vi "HFRR ADV v026 new software.vi"() -> ()   [LabVIEW 2025] (continued)
        n321 = Equal?(x=w400, y="Service@123") -> (x = y?=w401:bool)
        n322 = case shown="False" w401 {
          selector: w401 -> [w405 w407]
          frame False {
            n323 = local write "Service Password enable"(w405) -> ()
            n324 = property on="Service Password Log" class="Str"("Visible"=TRUE) -> ()  [unwired: 2 in, 2 out]
          }
          frame True {
            n325 = property on="Service Password Log" class="Str"("Visible"=FALSE) -> ()  [unwired: 2 in, 2 out]
            "Service Password enable" <- w407
          }
        }
      }
      event "Sign In": Value Change {
        w409 = FALSE ("Visible")
        n326 = event-data() -> ()  [unwired: 1 in, 6 out]
        n327 = property on="About" class="Clust (strict)"("Visible"=w409) -> ()  [unwired: 2 in, 2 out]
        n328 = property on="Password 3" class="Clust (strict)"("Visible"=w409) -> ()  [unwired: 2 in, 2 out]
        n329 = property on="Service Password Log" class="Str"("Visible"=FALSE) -> ()  [unwired: 2 in, 2 out]
      }
      event "Info": Value Change {
        n330 = event-data() -> ()  [unwired: 1 in, 6 out]
        n331 = local read "Info"() -> (w411:bool)
        n332 = case shown="False" w411 {
          frame False {
            n333 = property on="About" class="Clust (strict)"("Visible"=FALSE) -> ()  [unwired: 2 in, 2 out]
          }
          frame True {
            n334 = property on="About" class="Clust (strict)"("Visible"=TRUE) -> ()  [unwired: 2 in, 2 out]
          }
        }
      }
      event "Calibration": Value Change {
        n335 = event-data() -> ()  [unwired: 1 in, 6 out]
        n336 = local read "Calibration"() -> (w415:bool)
        n337 = case shown="False" w415 {
          frame False {
            n338 = property on="Calibration 2" class="TabCtl (strict)"("Visible"=FALSE) -> ()  [unwired: 2 in, 2 out]
            n339 = local write "Cal Password"("" ("Cal Password")) -> ()
          }
          frame True {
            n340 = property on="Calibration 2" class="TabCtl (strict)"("Visible"=TRUE) -> ()  [unwired: 2 in, 2 out]
            n341 = local write "Cal Password"("" ("Cal Password")) -> ()
          }
        }
        n342 = property on="Wrong Password" class="Str"("Visible"=FALSE) -> ()  [unwired: 2 in, 2 out]
      }
      event "Cal Password": Value Change {
        n343 = event-data() -> ()  [unwired: 1 in, 6 out]
        n344 = local read "Cal Password"() -> (w423:string)
        n345 = call <vilib>:"Trim Whitespace.vi"("string"=w423) -> ("trimmed string"=w422:string)  [unwired: 1 in]
        n346 = Equal?(x=w422, y="Cal@321") -> (x = y?=w420:bool)
        n347 = case shown="True" w420 {
          frame False {
            n348 = property on="Wrong Password" class="Str"("Visible"=TRUE) -> ()  [unwired: 2 in, 2 out]
          }
          frame True {
            n349 = property on="Wrong Password" class="Str"("Visible"=FALSE) -> ()  [unwired: 2 in, 2 out]
            n350 = local write "Main Tab"(T2."About" ("Main Tab")) -> ()
            n351 = local write "Cal Password"("" ("Cal Password")) -> ()
            n352 = local write "Main Dashboard Buttons"(T1."About" ("Main Dashboard Buttons")) -> ()
            n353 = property on="Calibration 2" class="TabCtl (strict)"("Visible"=FALSE) -> ()  [unwired: 2 in, 2 out]
            n354 = local write "Calibration"(FALSE ("Calibration")) -> ()
          }
        }
      }
      event "Calibration Selection": Value Change {
        n355 = event-data() -> ()  [unwired: 1 in, 6 out]
        n356 = local read "Calibration Selection"() -> (w432:T8)
        n357 = case shown="\"Stroke Calibration\"" w432 {
          tunnel: [T7."Stroke" ("Main Calibration Tab") T7."Friction" ("Main Calibration Tab") T7."Main" ("Main Calibration Tab") T7."Temperature" ("Main Calibration Tab")] -> w431
          frame "Stroke Calibration" {
          }
          frame "Friction Force Calibration" {
          }
          frame Default {
          }
          frame "Temperature Calibration" {
          }
        }
        n358 = local write "Main Calibration Tab"(w431) -> ()
      }
      event "Back Stroke": Value Change {
        n359 = event-data() -> ()  [unwired: 1 in, 6 out]
        n360 = local write "Main Stroke Tab"(T9."Step 1" ("Main Stroke Tab")) -> ()
        n361 = local write "Main Calibration Tab"(T7."Main" ("Main Calibration Tab")) -> ()
        n362 = local write "Back Stroke"(FALSE ("Back Stroke")) -> ()
      }
      event "Step 2 Back": Value Change {
        n363 = event-data() -> ()  [unwired: 1 in, 6 out]
        n364 = local write "Main Stroke Tab"(T9."Step 1" ("Main Stroke Tab")) -> ()
        n365 = local write "Step 2 Back"(FALSE ("Back Stroke")) -> ()
      }
      event "Step 3 Back": Value Change {
        n366 = event-data() -> ()  [unwired: 1 in, 6 out]
        n367 = local write "Main Stroke Tab"(T9."Step 2" ("Main Stroke Tab")) -> ()
        n368 = local write "Step 3 Back"(FALSE ("Back Stroke")) -> ()
      }
      event "Step 4 Back": Value Change {
        n369 = event-data() -> ()  [unwired: 1 in, 6 out]
        n370 = local write "Main Stroke Tab"(T9."Step 3" ("Main Stroke Tab")) -> ()
        n371 = local write "Step 4 Back"(FALSE ("Back Stroke")) -> ()
      }
      event "Step 5 Back": Value Change {
        n372 = event-data() -> ()  [unwired: 1 in, 6 out]
        n373 = local write "Main Stroke Tab"(T9."Step 4" ("Main Stroke Tab")) -> ()
        n374 = local write "Step 5 Back"(FALSE ("Back Stroke")) -> ()
      }
      event "Step 6 Back": Value Change {
        n375 = event-data() -> ()  [unwired: 1 in, 6 out]
        n376 = local write "Main Stroke Tab"(T9."Step 5" ("Main Stroke Tab")) -> ()
        n377 = local write "Step 6 Back"(FALSE ("Back Stroke")) -> ()
      }
      event "Back Stroke step 7": Value Change {
        n378 = event-data() -> ()  [unwired: 1 in, 6 out]
        n379 = local write "Main Stroke Tab"(T9."Step 6" ("Main Stroke Tab")) -> ()
        n380 = local write "Back Stroke step 7"(FALSE ("Back Stroke")) -> ()
      }
      event "Back Stroke step 8": Value Change {
        n381 = event-data() -> ()  [unwired: 1 in, 6 out]
        n382 = local write "Main Stroke Tab"(T9."Step 7" ("Main Stroke Tab")) -> ()
        n383 = local write "Back Stroke step 8"(FALSE ("Back Stroke")) -> ()
      }
      event "Back Stroke 8": Value Change {
        n384 = event-data() -> ()  [unwired: 1 in, 6 out]
        n385 = local write "MOVE CARRIAGE TO"(0.2 ("MOVE CARRIAGE TO")) -> ()
        n386 = local write "Main Stroke Tab"(T9."Step 1" ("Main Stroke Tab")) -> ()
        n387 = local write "Back Stroke 8"(FALSE ("Back Stroke 8")) -> ()
      }
      event "Continue Stroke": Value Change {
        n388 = event-data() -> ()  [unwired: 1 in, 6 out]
        n389 = local write "Main Stroke Tab"(T9."Step 2" ("Main Stroke Tab")) -> ()
        n390 = local write "Continue Stroke"(FALSE ("Continue Stroke")) -> ()
      }
      event "Continue Stroke step 2": Value Change {
        n391 = event-data() -> ()  [unwired: 1 in, 6 out]
        n392 = local write "Main Stroke Tab"(T9."Step 3" ("Main Stroke Tab")) -> ()
        n393 = local write "Continue Stroke step 2"(FALSE ("Continue Stroke")) -> ()
      }
      event "Continue Stroke step 3": Value Change {
        n394 = event-data() -> ()  [unwired: 1 in, 6 out]
        n395 = local write "Main Stroke Tab"(T9."Step 4" ("Main Stroke Tab")) -> ()
        n396 = local write "Continue Stroke step 3"(FALSE ("Continue Stroke")) -> ()
      }
      event "Continue Stroke step 4": Value Change {
        n397 = event-data() -> ()  [unwired: 1 in, 6 out]
        n398 = local write "Main Stroke Tab"(T9."Step 5" ("Main Stroke Tab")) -> ()
        n399 = local write "Continue Stroke step 4"(FALSE ("Continue Stroke")) -> ()
      }
      event "Continue Stroke step 5": Value Change {
        n400 = event-data() -> ()  [unwired: 1 in, 6 out]
        n401 = local write "Main Stroke Tab"(T9."Step 6" ("Main Stroke Tab")) -> ()
        n402 = local write "Continue Stroke step 5"(FALSE ("Continue Stroke")) -> ()
      }
      event "Continue Stroke step 6": Value Change {
        n403 = event-data() -> ()  [unwired: 1 in, 6 out]
        n404 = local write "Main Stroke Tab"(T9."Step 7" ("Main Stroke Tab")) -> ()
        n405 = local write "Continue Stroke step 6"(FALSE ("Continue Stroke")) -> ()
      }
      event "Continue Stroke step 7": Value Change {
        w471 = FALSE ("0.2mm")
        n406 = event-data() -> ()  [unwired: 1 in, 6 out]
        n407 = local write "0.4 mm"(w471) -> ()
        n408 = local write "0.6 mm"(w471) -> ()
        n409 = local write "1.0 mm"(w471) -> ()
        n410 = local write "1.2 mm"(w471) -> ()
        n411 = local write "0.2 2"(w471) -> ()
        n412 = local write "0.4 2"(w471) -> ()
        n413 = local write "0.6 2"(w471) -> ()
        n414 = local write "0.8 2"(w471) -> ()
        n415 = local write "1.0 2"(w471) -> ()
        n416 = local write "1.2"(w471) -> ()
        n417 = local write "0.2mm"(w471) -> ()
        n418 = local write "0.8mm"(w471) -> ()
        n419 = local write "Main Stroke Tab"(T9."Step 8" ("Main Stroke Tab")) -> ()
        n420 = local write "Continue Stroke step 7"(FALSE ("Continue Stroke")) -> ()
        n421 = local write "Stroke Test Complete"(T10."Test Progress" ("Stroke Test Complete")) -> ()
        "Position Measurment Temp" <- 0.0 ("Position Measurment Temp")
        "Calibration Tare" <- TRUE ("Calibration Tare")
        "MOVE CARRIAGE TO" <- 0.2 ("MOVE CARRIAGE TO")
      }
      event "Continue Stroke step 8": Value Change {
        n422 = event-data() -> ()  [unwired: 1 in, 6 out]
        n423 = local read "LVDT STROKE  Calibration"() -> (w476:dbl)
        n424 = local read "Position Measurment Temp"() -> (w477:dbl)
        n425 = case shown="7" w477 {
          selector: w477 -> [w482 w487 w492 w497 w502 w506 w509 w510]
          tunnel: w476 -> [w478 w483 w488 w493 w498 w503 _ _]
          frame 0, Default {
            w480 = TRUE ("0.2mm")
            n426 = Increment(x=w482) -> (x+1=w481:i32)
            n427 = local write "Position Measurment Temp"(w481) -> ()
            n428 = local write "0.2mm"(w480) -> ()
            n429 = local write "0.2 2"(w480) -> ()
            n430 = local write "MOVE CARRIAGE TO"(0.4 ("MOVE CARRIAGE TO")) -> ()
            "Calibration 0.2" <- w478
          }
          frame 1 {
            w485 = TRUE ("0.4 mm")
            n431 = Increment(x=w487) -> (x+1=w486:i32)
            n432 = local write "Calibration 0.4"(w483) -> ()
            n433 = local write "Position Measurment Temp"(w486) -> ()
            n434 = local write "0.4 mm"(w485) -> ()
            n435 = local write "MOVE CARRIAGE TO"(0.6 ("MOVE CARRIAGE TO")) -> ()
            n436 = local write "0.4 2"(w485) -> ()
          }
          frame 2 {
            w490 = TRUE ("0.6 mm")
            n437 = Increment(x=w492) -> (x+1=w491:i32)
            n438 = local write "Calibration 0.6"(w488) -> ()
            n439 = local write "Position Measurment Temp"(w491) -> ()
            n440 = local write "0.6 2"(w490) -> ()
            n441 = local write "0.6 mm"(w490) -> ()
            n442 = local write "MOVE CARRIAGE TO"(0.8 ("MOVE CARRIAGE TO")) -> ()
          }
          frame 3 {
            w494 = TRUE ("0.6 mm")
            n443 = Increment(x=w497) -> (x+1=w496:i32)
            n444 = local write "Position Measurment Temp"(w496) -> ()
            n445 = local write "MOVE CARRIAGE TO"(1.0 ("MOVE CARRIAGE TO")) -> ()
            n446 = local write "0.8mm"(w494) -> ()
            n447 = local write "0.8 2"(w494) -> ()
            "Calibration 0.8" <- w493
          }
          frame 4 {
            w499 = TRUE ("0.6 mm")
            n448 = Increment(x=w502) -> (x+1=w501:i32)
            n449 = local write "Position Measurment Temp"(w501) -> ()
            n450 = local write "MOVE CARRIAGE TO"(1.2 ("MOVE CARRIAGE TO")) -> ()
            n451 = local write "1.0 mm"(w499) -> ()
            n452 = local write "1.0 2"(w499) -> ()
            "Calibration 1.0" <- w498
          }
          frame 5 {
            w504 = TRUE ("0.6 mm")
            n453 = Increment(x=w506) -> (x+1=w505:i32)
            n454 = local write "Position Measurment Temp"(w505) -> ()
            n455 = local write "1.2 mm"(w504) -> ()
            n456 = local write "1.2"(w504) -> ()
            "Calibration 1.2" <- w503
          }
          frame 6 {
            n457 = Increment(x=w509) -> (x+1=w508:i32)
            n458 = local write "Position Measurment Temp"(w508) -> ()
            n459 = local write "Stroke Test Complete"(T10."Stroke Points Completed" ("Stroke Test Complete")) -> ()
          }
          frame 7 {
            n460 = stacked-sequence {
              tunnel: w510 -> [w511 _ _]
              frame #0 {
                n461 = Increment(x=w511) -> (x+1=w512:i32)
                n462 = local write "Main Stroke Tab"(T9."Step 9" ("Main Stroke Tab")) -> ()
                n463 = local write "Position Measurment Temp"(w512) -> ()
                n464 = Insert Into Array(array=dbl[] [], new element #1=0.2 ("new element/subarray"), new element #2=0.4 ("new element/subarray"), new element #3=0.6 ("new element/subarray"), new element #4=0.8 ("new element/subarray"), new element #5=1.0 ("new element/subarray"), new element #6=1.2 ("new element/subarray")) -> (→"1D stroke":dbl[])  [unwired: 1 in]
                n465 = local read "Calibration 0.2"() -> (w519:dbl)
                n466 = local read "Calibration 0.4"() -> (w518:dbl)
                n467 = local read "Calibration 0.6"() -> (w517:dbl)
                n468 = local read "Calibration 0.8"() -> (w516:dbl)
                n469 = local read "Calibration 1.0"() -> (w515:dbl)
                n470 = local read "Calibration 1.2"() -> (w514:dbl)
                n471 = Insert Into Array(array=dbl[] [], new element #1=w519, new element #2=w518, new element #3=w517, new element #4=w516, new element #5=w515, new element #6=w514) -> (→"Calibrated Voltage Value":dbl[])  [unwired: 1 in]
              }
              frame #1 {
                n472 = local read "calibration values"() -> (w542:dbl[])
                n473 = local read "Calibrated Voltage Value"() -> (w544:dbl[])
                n474 = Index Array(array=w542, index #1=1 ("index"), index #2=3 ("index"), index #3=5 ("index"), index #4=7 ("index"), index #5=9 ("index"), index #6=11 ("index")) -> (element #1=w535:dbl, element #2=w534:dbl, element #3=w533:dbl, element #4=w532:dbl, element #5=w531:dbl, element #6=w530:dbl)
                n475 = local read "1D stroke"() -> (w545:dbl[])
                n476 = for {
                  tunnel: [w554] -> w543 mode=indexing
                  tunnel: w545 -> [w553] mode=indexing
                  tunnel: w544 -> [w552] mode=indexing
                  tunnel: w535 -> [w551]
                  tunnel: w534 -> [w550]
                  tunnel: w533 -> [w549]
                  tunnel: w532 -> [w548]
                  tunnel: w531 -> [w547]
                  tunnel: w530 -> [w546]
                  n477 = formula code="if (stroke == 0.2)\n{\n    if ((voltage >= REF_02 - 0.2) && (voltage <= REF_02 + 0.2))\n        status = 1;\n    else\n        status = 0;\n}\nelse if (stroke == 0.4)\n{\n    if ((voltage >= REF_04 - 0.2) && (voltage <= REF_04 + 0.2))\n        status = 1;\n    else\n        status = 0;\n}\nelse if (stroke == 0.6)\n{\n    if ((voltage >= REF_06 - 0.2) && (voltage <= REF_06 + 0.2))\n        status = 1;\n    else\n        status = 0;\n}\nelse if (stroke == 0.8)\n{\n    if ((voltage >= REF_08 - 0.2) && (voltage <= REF_08 + 0.2))\n        status = 1;\n    else\n        status = 0;\n}\nelse if (stroke == 1.0)\n{\n    if ((voltage >= REF_10 - 0.2) && (voltage <= REF_10 + 0.2))\n        status = 1;\n    else\n        status = 0;\n}\nelse if (stroke == 1.2)\n{\n    if ((voltage >= REF_12 - 0.2) && (voltage <= REF_12 + 0.2))\n        status = 1;\n    else\n        status = 0;\n}\nelse\n{\n    status = 0;\n}"("stroke"=w553, "voltage"=w552, "REF_02"=w551, "REF_04"=w550, "REF_06"=w549, "REF_08"=w548, "REF_10"=w547, "REF_12"=w546) -> ("status"=w554:dbl)
                }
                "Status" <- w543
              }
              frame #2 {
                w561 = 1.0
                n478 = local read "Status"() -> (w568:dbl[])
                n479 = Index Array(array=w568) -> (element #1=w567:dbl, element #2=w566:dbl, element #3=w565:dbl, element #4=w564:dbl, element #5=w563:dbl, element #6=w562:dbl)  [unwired: 6 in]
                n480 = Equal?(x=w566, y=w561) -> (x = y?=w559:bool)
                n481 = Equal?(x=w565, y=w561) -> (x = y?=w558:bool)
                n482 = Equal?(x=w564, y=w561) -> (x = y?=w557:bool)
                n483 = Equal?(x=w563, y=w561) -> (x = y?=w556:bool)
                n484 = Equal?(x=w562, y=w561) -> (x = y?=w555:bool)
                n485 = Equal?(x=w567, y=w561) -> (x = y?=w560:bool)
                n486 = case shown="True" w560 {
                  selector: w560 -> [w579 w580]
                  frame True {
                    n487 = local write "Point 1 - 0.2 mm"(w579) -> ()
                    n488 = property on="Point 1 - 0.2 mm" class="Bool"("Caption.Visible"=w579) -> ()  [unwired: 2 in, 2 out]
                  }
                  frame False {
                    n489 = local write "Point 1 - 0.2 mm"(w580) -> ()
                    n490 = property on="Point 1 - 0.2 mm" class="Bool"("Caption.Visible"=w580) -> ()  [unwired: 2 in, 2 out]
                  }
                }
                n491 = case shown="True" w559 {
                  selector: w559 -> [w577 w578]
                  frame True {
                    n492 = local write "Point 2 - 0.4 mm"(w577) -> ()
                    n493 = property on="Point 2 - 0.4 mm" class="Bool"("Caption.Visible"=w577) -> ()  [unwired: 2 in, 2 out]
                  }
                  frame False {
                    n494 = local write "Point 2 - 0.4 mm"(w578) -> ()
                    n495 = property on="Point 2 - 0.4 mm" class="Bool"("Caption.Visible"=w578) -> ()  [unwired: 2 in, 2 out]
                  }
                }
                n496 = case shown="True" w556 {
                  selector: w556 -> [w571 w572]
                  frame True {
                    n497 = local write "Point 5 - 1.0 mm"(w571) -> ()
                    n498 = property on="Point 5 - 1.0 mm" class="Bool"("Caption.Visible"=w571) -> ()  [unwired: 2 in, 2 out]
                  }
                  frame False {
                    n499 = local write "Point 5 - 1.0 mm"(w572) -> ()
                    n500 = property on="Point 5 - 1.0 mm" class="Bool"("Caption.Visible"=w572) -> ()  [unwired: 2 in, 2 out]
                  }
                }
                n501 = case shown="True" w558 {
                  selector: w558 -> [w575 w576]
                  frame True {
                    n502 = local write "Point 3 - 0.6 mm"(w575) -> ()
                    n503 = property on="Point 3 - 0.6 mm" class="Bool"("Caption.Visible"=w575) -> ()  [unwired: 2 in, 2 out]
                  }
                  frame False {
                    n504 = local write "Point 3 - 0.6 mm"(w576) -> ()
                    n505 = property on="Point 3 - 0.6 mm" class="Bool"("Caption.Visible"=w576) -> ()  [unwired: 2 in, 2 out]
                  }
                }
                n506 = case shown="True" w557 {
                  selector: w557 -> [w573 w574]
                  frame True {
                    n507 = local write "Point 4 - 0.8 mm"(w573) -> ()
                    n508 = property on="Point 4 - 0.8 mm" class="Bool"("Caption.Visible"=w573) -> ()  [unwired: 2 in, 2 out]
                  }
                  frame False {
                    n509 = local write "Point 4 - 0.8 mm"(w574) -> ()
                    n510 = property on="Point 4 - 0.8 mm" class="Bool"("Caption.Visible"=w574) -> ()  [unwired: 2 in, 2 out]
                  }
                }
                n511 = case shown="True" w555 {
                  selector: w555 -> [w569 w570]
                  frame True {
                    n512 = local write "Point 6 - 1.2 mm"(w569) -> ()
                    n513 = property on="Point 6 - 1.2 mm" class="Bool"("Caption.Visible"=w569) -> ()  [unwired: 2 in, 2 out]
                  }
                  frame False {
                    n514 = local write "Point 6 - 1.2 mm"(w570) -> ()
                    n515 = property on="Point 6 - 1.2 mm" class="Bool"("Caption.Visible"=w570) -> ()  [unwired: 2 in, 2 out]
                  }
                }
              }
            }
          }
        }
      }
      event "TEMPERATURE STEP Back 1", "TEMPERATURE STEP Back air Temp": Value Change {
        n516 = event-data() -> ()  [unwired: 1 in, 6 out]
        n517 = stacked-sequence {
          frame #0 {
            n518 = local write "Main Calibration Tab"(T7."Main" ("Main Calibration Tab")) -> ()
          }
          frame #1 {
            n519 = Wait (ms)(milliseconds to wait=u32 1000) -> ()  [unwired: 1 out]
          }
          frame #2 {
            n520 = local write "Due Write"("CAL;END" ("Command")) -> ()
          }
          frame #3 {
            n521 = Wait (ms)(milliseconds to wait=u32 2000) -> ()  [unwired: 1 out]
          }
          frame #4 {
            n522 = local write "Due Write"("CAL;END" ("Command")) -> ()
          }
        }
      }
      event "Temperature Continue Step 1": Value Change {
        n523 = event-data() -> ()  [unwired: 1 in, 6 out]
        n524 = stacked-sequence {
          frame #0 {
            n525 = Wait (ms)(milliseconds to wait=u32 1500) -> ()  [unwired: 1 out]
          }
          frame #1 {
            n526 = local write "Due Write"("CAL;START" ("Command")) -> ()
          }
          frame #2 {
            n527 = Wait (ms)(milliseconds to wait=u32 1500) -> ()  [unwired: 1 out]
          }
          frame #3 {
            n528 = local write "Due Write"("CAL;START" ("Command")) -> ()
          }
          frame #4 {
            n529 = Wait (ms)(milliseconds to wait=u32 2000) -> ()  [unwired: 1 out]
          }
          frame #5 {
          }
          frame #6 {
            n530 = Wait (ms)(milliseconds to wait=u32 2000) -> ()  [unwired: 1 out]
          }
          frame #7 {
            # "CAL;A1;<true_T>"
            n531 = local write "Due Write"("CAL;A1;0" ("Command")) -> ()
          }
          frame #8 {
            n532 = local write "Tab Control 4"(T11."Step 2" ("Tab Control 4")) -> ()
          }
        }
      }
      event "Temperature Continue Step air Step 1": Value Change {
        n533 = event-data() -> ()  [unwired: 1 in, 6 out]
        n534 = stacked-sequence {
          frame #0 {
            n535 = Wait (ms)(milliseconds to wait=u32 1500) -> ()  [unwired: 1 out]
          }
          frame #1 {
            n536 = local write "Due Write"("CAL;START" ("Command")) -> ()
          }
          frame #2 {
            n537 = Wait (ms)(milliseconds to wait=u32 1500) -> ()  [unwired: 1 out]
          }
          frame #3 {
            n538 = local write "Due Write"("CAL;START" ("Command")) -> ()
          }
          frame #4 {
            n539 = Wait (ms)(milliseconds to wait=u32 2000) -> ()  [unwired: 1 out]
          }
          frame #5 {
          }
          frame #6 {
            n540 = Wait (ms)(milliseconds to wait=u32 2000) -> ()  [unwired: 1 out]
          }
          frame #7 {
            # "CAL;A1;<true_T>"
            n541 = local write "Due Write"("CAL;A1;0" ("Command")) -> ()
          }
          frame #8 {
            n542 = local write "Tab Control 4"(T11."Air Step 2" ("Tab Control 4")) -> ()
          }
        }
      }
      event "Temperature Selection": Value Change {
        n543 = event-data() -> ()  [unwired: 1 in, 6 out]
        n544 = local read "Temperature Selection"() -> (w602:T12)
        n545 = case shown="\"Default\", Default" w602 {
          frame "Air Temperature" {
            n546 = local write "Tab Control 4"(T11."Air Step 1" ("Tab Control 4")) -> ()
          }
          frame "Sample Temperature" {
            n547 = local write "Tab Control 4"(T11."Step 1" ("Tab Control 4")) -> ()
          }
          frame "Default", Default {
          }
        }
      }
      event "Temperature Continue Step 2": Value Change {
        n548 = event-data() -> ()  [unwired: 1 in, 6 out]
        n549 = stacked-sequence {
          frame #0 {
            n550 = stacked-sequence {
              frame #0 {
                n551 = Wait (ms)(milliseconds to wait=u32 1500) -> ()  [unwired: 1 out]
              }
              frame #1 {
                # "CAL;A1;<true_T>"
                n552 = local write "Due Write"("CAL;A1;0" ("Command")) -> ()
              }
              frame #2 {
                n553 = Wait (ms)(milliseconds to wait=u32 1500) -> ()  [unwired: 1 out]
              }
              frame #3 {
                # "CAL;A1;<true_T>"
                n554 = local write "Due Write"("CAL;A1;0" ("Command")) -> ()
              }
              frame #4 {
              }
            }
          }
          frame #1 {
            n555 = local write "Tab Control 4"(T11."Step 3" ("Tab Control 4")) -> ()
          }
        }
      }
      event "Temperature Continue Step 5": Value Change {
        n556 = event-data() -> ()  [unwired: 1 in, 6 out]
        n557 = stacked-sequence {
          frame #0 {
            n558 = stacked-sequence {
              frame #0 {
                n559 = Wait (ms)(milliseconds to wait=u32 1500) -> ()  [unwired: 1 out]
              }
              frame #1 {
                # "CAL;A1;<true_T>"
                n560 = local write "Due Write"("CAL;A1;0" ("Command")) -> ()
              }
              frame #2 {
                n561 = Wait (ms)(milliseconds to wait=u32 1500) -> ()  [unwired: 1 out]
              }
              frame #3 {
                # "CAL;A1;<true_T>"
                n562 = local write "Due Write"("CAL;A1;0" ("Command")) -> ()
              }
              frame #4 {
              }
            }
          }
          frame #1 {
            n563 = local write "Tab Control 4"(T11."Air Step 3" ("Tab Control 4")) -> ()
          }
        }
      }
      event "Temperature Continue Step 3": Value Change {
        n564 = event-data() -> ()  [unwired: 1 in, 6 out]
        n565 = stacked-sequence {
          frame #0 {
            n566 = stacked-sequence {
              frame #0 {
                n567 = Wait (ms)(milliseconds to wait=u32 1500) -> ()  [unwired: 1 out]
              }
              frame #1 {
              }
              frame #2 {
              }
              frame #3 {
                # "CAL;A1;<true_T>"
                n568 = local write "Due Write"("CAL;A1;60" ("Command")) -> ()
              }
              frame #4 {
                n569 = Wait (ms)(milliseconds to wait=u32 2000) -> ()  [unwired: 1 out]
              }
              frame #5 {
                # "CAL;A1;<true_T>"
                n570 = local write "Due Write"("CAL;A1;60" ("Command")) -> ()
              }
            }
          }
          frame #1 {
            n571 = Wait (ms)(milliseconds to wait=u32 1000) -> ()  [unwired: 1 out]
          }
          frame #2 {
            n572 = local write "Due Write"("CAL;SAVE" ("Command")) -> ()
          }
          frame #3 {
            n573 = Wait (ms)(milliseconds to wait=u32 1000) -> ()  [unwired: 1 out]
          }
          frame #4 {
            n574 = local write "Due Write"("CAL;SAVE" ("Command")) -> ()
          }
          frame #5 {
            n575 = Wait (ms)(milliseconds to wait=u32 1000) -> ()  [unwired: 1 out]
          }
          frame #6 {
            # "CAL;END"
            n576 = local write "Due Write"("CAL;END" ("Command")) -> ()
          }
          frame #7 {
            n577 = Wait (ms)(milliseconds to wait=u32 1000) -> ()  [unwired: 1 out]
          }
          frame #8 {
            # "CAL;END"
            n578 = local write "Due Write"("CAL;END" ("Command")) -> ()
          }
          frame #9 {
            n579 = local write "Main Calibration Tab"(T7."Temperature" ("Main Calibration Tab")) -> ()
            n580 = local write "Tab Control 4"(T11."Main" ("Tab Control 4")) -> ()
          }
        }
      }
      event "Temperature Continue Step 6": Value Change {
        n581 = event-data() -> ()  [unwired: 1 in, 6 out]
        n582 = stacked-sequence {
          frame #0 {
            n583 = stacked-sequence {
              frame #0 {
                n584 = Wait (ms)(milliseconds to wait=u32 1500) -> ()  [unwired: 1 out]
              }
              frame #1 {
              }
              frame #2 {
              }
              frame #3 {
                # "CAL;A1;<true_T>"
                n585 = local write "Due Write"("CAL;A1;60" ("Command")) -> ()
              }
              frame #4 {
                n586 = Wait (ms)(milliseconds to wait=u32 2000) -> ()  [unwired: 1 out]
              }
              frame #5 {
                # "CAL;A1;<true_T>"
                n587 = local write "Due Write"("CAL;A1;60" ("Command")) -> ()
              }
            }
          }
          frame #1 {
            n588 = Wait (ms)(milliseconds to wait=u32 1000) -> ()  [unwired: 1 out]
          }
          frame #2 {
            n589 = local write "Due Write"("CAL;SAVE" ("Command")) -> ()
          }
          frame #3 {
            n590 = Wait (ms)(milliseconds to wait=u32 1000) -> ()  [unwired: 1 out]
          }
          frame #4 {
            n591 = local write "Due Write"("CAL;SAVE" ("Command")) -> ()
          }
          frame #5 {
            n592 = Wait (ms)(milliseconds to wait=u32 1000) -> ()  [unwired: 1 out]
          }
          frame #6 {
            # "CAL;END"
            n593 = local write "Due Write"("CAL;END" ("Command")) -> ()
          }
          frame #7 {
            n594 = Wait (ms)(milliseconds to wait=u32 1000) -> ()  [unwired: 1 out]
          }
          frame #8 {
            # "CAL;END"
            n595 = local write "Due Write"("CAL;END" ("Command")) -> ()
          }
          frame #9 {
            n596 = local write "Main Calibration Tab"(T7."Temperature" ("Main Calibration Tab")) -> ()
            n597 = local write "Tab Control 4"(T11."Main" ("Tab Control 4")) -> ()
          }
        }
      }
      event "Back Stroke step main temperature": Value Change {
        n598 = event-data() -> ()  [unwired: 1 in, 6 out]
        n599 = stacked-sequence {
          frame #0 {
            n600 = Wait (ms)(milliseconds to wait=u32 1000) -> ()  [unwired: 1 out]
          }
          frame #1 {
            # "CAL;END"
            n601 = local write "Due Write"("CAL;END" ("Command")) -> ()
          }
          frame #2 {
            n602 = Wait (ms)(milliseconds to wait=u32 1000) -> ()  [unwired: 1 out]
          }
          frame #3 {
            # "CAL;END"
            n603 = local write "Due Write"("CAL;END" ("Command")) -> ()
          }
          frame #4 {
            n604 = local write "Main Calibration Tab"(T7."Temperature" ("Main Calibration Tab")) -> ()
            n605 = local write "Tab Control 4"(T11."Main" ("Tab Control 4")) -> ()
          }
        }
      }
      event "TEMPERATURE STEP  Back 4", "TEMPERATURE STEP 1 Back 3", "TEMPERATURE STEP  Back 3", "TEMPERATURE STEP 1 Back 2": Value Change {
        n606 = event-data() -> ()  [unwired: 1 in, 6 out]
        n607 = stacked-sequence {
          frame #0 {
            n608 = Wait (ms)(milliseconds to wait=u32 1000) -> ()  [unwired: 1 out]
          }
          frame #1 {
            # "CAL;END"
            n609 = local write "Due Write"("CAL;END" ("Command")) -> ()
          }
          frame #2 {
            n610 = Wait (ms)(milliseconds to wait=u32 1000) -> ()  [unwired: 1 out]
          }
          frame #3 {
            # "CAL;END"
            n611 = local write "Due Write"("CAL;END" ("Command")) -> ()
          }
          frame #4 {
            # "TEMPERATURE STEP  Back 4"
            n612 = local write "Main Calibration Tab"(T7."Temperature" ("Main Calibration Tab")) -> ()
            n613 = local write "Tab Control 4"(T11."Main" ("Tab Control 4")) -> ()
          }
        }
      }
      event "Quit": Value Change {
        n614 = event-data() -> ()  [unwired: 1 in, 6 out]
      }
    }
    n615 = Wait (ms)(milliseconds to wait=u32 100) -> ()  [unwired: 1 out]
  }
  n616 = while {
    stop <- w672 stop-if-true
    n617 = local read "Ambient Temperature"() -> (w670:dbl)
    n618 = local read "Sample Temperature"() -> (w669:dbl)
    n619 = Wait (ms)(milliseconds to wait=u32 200) -> ()  [unwired: 1 out]
    n620 = local write "Temperature — Live (Set A: 0 °C)"(w670) -> ()
    n621 = local write "Temperature — Live (Set A: 60 °C)"(w670) -> ()
    n622 = local write "Sensor value"(w670) -> ()
    n623 = local write "Sensor value"(w670) -> ()
    n624 = local write "Sensor value"(w669) -> ()
    n625 = local write "Sensor value"(w669) -> ()
    n626 = local write "Temperature — Live (Set A: 60 °C)"(w669) -> ()
    n627 = local write "Temperature — Live (Set A: 0 °C)"(w669) -> ()
    n628 = case shown="True" "Save Button" {
      selector: "Save Button" -> [_ w678]
      frame False {
      }
      frame True {
        n629 = Not(x=w678) -> (.not. x?=w677:bool)
        n630 = local read "milliseconds to wait"() -> (w710:u32)
        n631 = local read "max_step_change"() -> (w715:dbl)
        n632 = local read "max_amplitude"() -> (w716:dbl)
        n633 = local read "min_amplitude"() -> (w717:dbl)
        n634 = local read "PIEZO_CAL_FACTOR"() -> (w721:dbl)
        n635 = local write "Save Button"(w677) -> ()
        n636 = local read "startup_cmd"() -> (w718:dbl)
        n637 = local read "NORMAL_FORCE"() -> (w722:dbl)
        n638 = local read "ADC_Resolution"() -> (w720:dbl)
        n639 = local read "calibration values"() -> (w725:dbl[])
        n640 = local read "kp"() -> (w712:dbl)
        n641 = local read "kd"() -> (w714:dbl)
        n642 = local read "dt"() -> (w711:dbl)
        n643 = local read "ki"() -> (w713:dbl)
        n644 = local read "STROKE FILTER"() -> (w723:i32)
        n645 = local read "Add up Stroke"() -> (w724:dbl)
        n646 = local read "VREF"() -> (w719:dbl)
        n647 = Insert Into Array(array=dbl[] [], new element #1=w710, new element #2=w711, new element #3=w712, new element #4=w713, new element #5=w714, new element #6=w715, new element #7=w716, new element #8=w717, new element #9=w718) -> (w726:dbl[])  [unwired: 1 in]
        n648 = Insert Into Array(array=dbl[] [], new element #1=w719, new element #2=w720, new element #3=w721, new element #4=w722) -> (w727:dbl[])  [unwired: 1 in]
        n649 = Array To Spreadsheet String(delimiter (Tab)=";", array=w725, 3:"" ("format string")) -> (spreadsheet string=w729:string)
        n650 = Insert Into Array(array=dbl[] [], new element #1=w723, new element #2=w724) -> (w728:dbl[])  [unwired: 1 in]
        n651 = call "Write Config.vi"("Stroke Calibration"=w729, "STROKE PARAMETERS"=w728, "ADC PARAMETERS"=w727, "PID  PARAMETERS"=w726) -> ("error out"=w708:errorcluster)  [unwired: 7 in]
        n652 = call "Stall Data Flow.vim"("value in"=w708, "milliseconds to wait"=u32 2000) -> ("value out"=w709:errorcluster)  [unwired: 1 out]
        n653 = call "Read Config.vi"("error in (no error)"=w709) -> ("STROKE PARAMETERS"=w706:dbl[], "ADC PARAMETERS"=w705:dbl[], "PID  PARAMETERS"=w704:dbl[], "Stroke Calibration"=w707:string)  [unwired: 6 in, 1 out]
        n654 = Index Array(array=w704) -> (element #1=w702:dbl, element #2=w701:dbl, element #3=w700:dbl, element #4=w699:dbl, element #5=w698:dbl, element #6=w697:dbl, element #7=w696:dbl, element #8=w695:dbl, element #9=w694:dbl)  [unwired: 9 in]
        n655 = Index Array(array=w705) -> (element #1=w693:dbl, element #2=w692:dbl, element #3=w691:dbl, element #4=w690:dbl)  [unwired: 4 in]
        n656 = Index Array(array=w706) -> (element #1=w689:dbl, element #2=w688:dbl)  [unwired: 2 in]
        n657 = Spreadsheet String To Array(delimiter (Tab)=";", format string="", spreadsheet string=w707, array type (2D Dbl)=dbl[] []) -> (array=w703:dbl[])
        n658 = local write "VREF"(w693) -> ()
        n659 = local write "ADC_Resolution"(w692) -> ()
        n660 = local write "PIEZO_CAL_FACTOR"(w691) -> ()
        n661 = local write "NORMAL_FORCE"(w690) -> ()
        n662 = local write "STROKE FILTER"(w689) -> ()
        n663 = local write "Add up Stroke"(w688) -> ()
        n664 = local write "calibration values"(w703) -> ()
        n665 = local write "milliseconds to wait"(w702) -> ()
        n666 = local write "dt"(w701) -> ()
        n667 = local write "kp"(w700) -> ()
        n668 = local write "ki"(w699) -> ()
        n669 = local write "kd"(w698) -> ()
        n670 = local write "max_step_change"(w697) -> ()
        n671 = local write "max_amplitude"(w696) -> ()
        n672 = local write "min_amplitude"(w695) -> ()
        n673 = local write "startup_cmd"(w694) -> ()
      }
    }
    n674 = local read "USER ID"() -> (w667:string)
    n675 = local write "tested by 2"(w667) -> ()
    n676 = local read "Point 1 - 0.2 mm"() -> (w666:bool)
    n677 = local read "Point 2 - 0.4 mm"() -> (w665:bool)
    n678 = local read "Point 3 - 0.6 mm"() -> (w664:bool)
    n679 = local read "Point 4 - 0.8 mm"() -> (w663:bool)
    n680 = local read "Point 5 - 1.0 mm"() -> (w662:bool)
    n681 = local read "Point 6 - 1.2 mm"() -> (w661:bool)
    n682 = And(x=w666, y=w665) -> (x .and. y?=w660:bool)
    n683 = And(x=w664, y=w663) -> (x .and. y?=w659:bool)
    n684 = And(x=w662, y=w661) -> (x .and. y?=w657:bool)
    n685 = And(x=w660, y=w659) -> (x .and. y?=w658:bool)
    n686 = And(x=w658, y=w657) -> (x .and. y?=w656:bool)
    n687 = case shown="False" w656 {
      frame False {
        n688 = property on="Accept & Save" class="Bool (strict)"("DisabledEnum"=T18."Disabled" ("Disabled")) -> ()  [unwired: 2 in, 2 out]
        n689 = property on="Tab Control 5" class="TabCtl (strict)"("Value"=enum32{"OK", "NG"}."NG" ("Tab Control 5")) -> ()  [unwired: 2 in, 2 out]
      }
      frame True {
        n690 = property on="Accept & Save" class="Bool (strict)"("DisabledEnum"=T18."Enabled" ("Disabled")) -> ()  [unwired: 2 in, 2 out]
        n691 = property on="Tab Control 5" class="TabCtl (strict)"("Value"=enum32{"OK", "NG"}."OK" ("Tab Control 5")) -> ()  [unwired: 2 in, 2 out]
      }
    }
    n692 = local read "Quit"() -> (w672:bool)
  }
  n693 = while {
    shift-right: [w731] -> _
    shift-left: "Enum - Selector" -> [w732]
    stop <- w733 stop-if-true
    # "Auto Start Logic Loop"
    n694 = case shown="\"Humidity & Temperature On\"" w732 {
      tunnel: [w736 w742 w769 w801 w831 Auto_Start_enum."Exit" ("Enum - Selector") Auto_Start_enum."Init" ("Enum - Selector")] -> w731
      frame "Init", Default {
        n695 = local read "Auto Start Test"() -> (w735:bool)
        n696 = Select(t=Auto_Start_enum."Humidity & Temperature On" ("Enum - Selector"), s=w735, f=Auto_Start_enum."Init") -> (s? t:f=w736:T14)
      }
      frame "Humidity & Temperature On" {
        n697 = stacked-sequence {
          tunnel: [_ _ _ _ _ _ Auto_Start_enum."Reach point" ("Enum - Selector")] -> w739
          frame #0 {
            w744 = T18."Disabled and Grayed Out" ("Disabled")
            w745 = TRUE ("Heater Button")
            n698 = property on="Humidity" class="Bool (strict)"("DisabledEnum"=w744) -> ()  [unwired: 2 in, 2 out]
            n699 = property on="Heater Button" class="Bool (strict)"("DisabledEnum"=w744) -> ()  [unwired: 2 in, 2 out]
            n700 = local write "Heater Button"(w745) -> ()
            n701 = local write "Humidity"(w745) -> ()
            n702 = property on="Heater Button" class="Bool (strict)"("Val(Sgnl)"=TRUE ("Value (Signaling)")) -> ()  [unwired: 2 in, 2 out]
          }
          frame #1 {
            n703 = Wait (ms)(milliseconds to wait=u32 3000) -> ()  [unwired: 1 out]
          }
          frame #2 {
            n704 = local read "Set Temp"() -> (w751:dbl)
            n705 = Number To Fractional String(number=w751, precision (6)=i16 2) -> (F-format string=w748:string)  [unwired: 2 in]
            n706 = Concatenate Strings("ST;" ("Command"), w748) -> (w749:string)
            n707 = local write "Due Write"(w749) -> ()
          }
          frame #3 {
            n708 = Wait (ms)(milliseconds to wait=u32 1500) -> ()  [unwired: 1 out]
          }
          frame #4 {
            (unwired) i16 2 ("precision (6)")
            n709 = local read "Write UNO"() -> (w753:string[])
            n710 = local read "Set Rh"() -> (w756:dbl)
            n711 = Number To Fractional String(number=w756) -> (F-format string=w757:string)  [unwired: 3 in]
            n712 = Concatenate Strings("M;" ("new element/subarray"), w757) -> (w758:string)
            n713 = local write "Due Write"("HE;1" ("Command")) -> ()
            n714 = Insert Into Array(array=w753, new element=w758) -> (w754:string[])  [unwired: 1 in]
            n715 = local write "Write UNO"(w754) -> ()
          }
          frame #5 {
            n716 = Wait (ms)(milliseconds to wait=u32 1500) -> ()  [unwired: 1 out]
          }
          frame #6 {
            w761 = TRUE ("Reach point temp")
            n717 = local write "Reach point Humidity"(w761) -> ()
            n718 = local write "Reach point temp"(w761) -> ()
          }
        }
        n719 = local read "Auto Start Test"() -> (w741:bool)
        n720 = Not(x=w741) -> (.not. x?=w740:bool)
        n721 = Select(t=Auto_Start_enum."close", s=w740, f=w739) -> (s? t:f=w742:T14)
      }
      frame "Reach point" {
        w770 = TRUE ("PAUSE")
        w778 = 1.0 ("y")
        w781 = 1.0 ("y")
        n722 = local read "Set Temp"() -> (w763:dbl)
        n723 = local read "Set Humidity:"() -> (w777:dbl)
        n724 = local read "Humidity ( %RH )"() -> (w782:dbl)
        n725 = Add(x=w763, y=w781) -> (x+y=w780:dbl)
        n726 = Subtract(x=w763, y=w781) -> (x-y=w779:dbl)
        n727 = Add(x=w777, y=w778) -> (x+y=w776:dbl)
        n728 = Subtract(x=w777, y=w778) -> (x-y=w775:dbl)
        n729 = local read "TEMP"() -> (w783:dbl)
        n730 = In Range and Coerce(upper limit=w776, x=w782, lower limit=w775) -> (In Range?=w764:bool)  [unwired: 1 out]
        n731 = In Range and Coerce(upper limit=w780, x=w783, lower limit=w779) -> (In Range?=w765:bool)  [unwired: 1 out]
        n732 = case shown="True" w764 {
          frame False {
          }
          frame True {
            n733 = case shown="True" "Reach point Humidity" {
              selector: "Reach point Humidity" -> [_ w789]
              frame False {
              }
              frame True {
                n734 = local read "EVENT LOG"() -> (w786:string)
                n735 = Not(x=w789) -> (.not. x?=w788:bool)
                n736 = local write "Reach point Humidity"(w788) -> ()
                n737 = call "Event Log.vi"("Content"="Target Humidity reached", "EVENT LOG"=w786) -> ("EVENT LOG"=w787:string)  [unwired: 8 in, 1 out]
                n738 = local write "EVENT LOG"(w787) -> ()
              }
            }
          }
        }
        n739 = case shown="True" w765 {
          frame False {
          }
          frame True {
            n740 = case shown="True" "Reach point temp" {
              selector: "Reach point temp" -> [_ w795]
              frame False {
              }
              frame True {
                n741 = local read "EVENT LOG"() -> (w792:string)
                n742 = Not(x=w795) -> (.not. x?=w794:bool)
                n743 = local write "Reach point temp"(w794) -> ()
                n744 = call "Event Log.vi"("Content"="Target Temperature reached", "EVENT LOG"=w792) -> ("EVENT LOG"=w793:string)  [unwired: 8 in, 1 out]
                n745 = local write "EVENT LOG"(w793) -> ()
              }
            }
          }
        }
        n746 = local read "Auto Start Test"() -> (w768:bool)
        n747 = And(x=w765, y=w764) -> (x .and. y?=w774:bool)
        n748 = Select(t=Auto_Start_enum."Maintain Stage" ("Enum - Selector"), s=w774, f=Auto_Start_enum."Reach point" ("Enum - Selector")) -> (s? t:f=w771:T14)
        n749 = Not(x=w768) -> (.not. x?=w767:bool)
        n750 = Select(t=Auto_Start_enum."close", s=w767, f=w771) -> (s? t:f=w769:T14)
        n751 = call "ELAPSED TIMER VI.vi"("RESET"=w770, "PAUSE"=w770) -> ()  [unwired: 7 in, 3 out]
      }
      frame "Maintain Stage" {
        w810 = 2.0 ("y")
        w809 = 1.0 ("y")
        # "Humidity and  temperatures Set Point  have been reached"
        n752 = local read "Set Temp"() -> (w796:dbl)
        n753 = local read "Set Humidity:"() -> (w813:dbl)
        n754 = local read "Humidity ( %RH )"() -> (w816:dbl)
        n755 = Add(x=w796, y=w809) -> (x+y=w815:dbl)
        n756 = Subtract(x=w796, y=w809) -> (x-y=w814:dbl)
        n757 = local read "TEMP"() -> (w817:dbl)
        n758 = Add(x=w813, y=w810) -> (x+y=w812:dbl)
        n759 = Subtract(x=w813, y=w810) -> (x-y=w811:dbl)
        n760 = In Range and Coerce(upper limit=w815, x=w817, lower limit=w814) -> (In Range?=w808:bool)  [unwired: 1 out]
        n761 = In Range and Coerce(upper limit=w812, x=w816, lower limit=w811) -> (In Range?=w807:bool)  [unwired: 1 out]
        n762 = And(x=w808, y=w807) -> (x .and. y?=w806:bool)
        n763 = Not(x=w806) -> (.not. x?=w805:bool)
        n764 = call "ELAPSED TIMER VI.vi"("TARGET"=60.0, "RESET"=w805, "PAUSE"=FALSE) -> ("ELAPSED INDICATION"=w802:bool)  [unwired: 6 in, 2 out]
        n765 = case shown="True" w802 {
          tunnel: w802 -> [_ w820]
          tunnel: [Auto_Start_enum."Maintain Stage" ("Enum - Selector") w819] -> w800
          frame False {
          }
          frame True {
            n766 = stacked-sequence {
              tunnel: w820 -> [_ _ _ _ _]
              tunnel: [_ _ _ _ Auto_Start_enum."Start Stage" ("Enum - Selector")] -> w819
              frame #0 {
                n767 = local read "EVENT LOG"() -> (w822:string)
                n768 = call "Event Log.vi"("Content"="Humidity and temperature set point has stabilized.", "EVENT LOG"=w822) -> ("EVENT LOG"=w823:string)  [unwired: 8 in, 1 out]
                n769 = local write "EVENT LOG"(w823) -> ()
              }
              frame #1 {
                n770 = Wait (ms)(milliseconds to wait=u32 100) -> ()  [unwired: 1 out]
              }
              frame #2 {
                n771 = local read "EVENT LOG"() -> (w826:string)
                n772 = call "Event Log.vi"("Content"="Auto Test Started", "EVENT LOG"=w826) -> ("EVENT LOG"=w827:string)  [unwired: 8 in, 1 out]
                n773 = local write "EVENT LOG"(w827) -> ()
              }
              frame #3 {
                w828 = TRUE ("RUN")
                n774 = local write "RUN"(w828) -> ()
                n775 = property on="Auto Start Temp" class="Bool (strict)"("Val(Sgnl)"=w828) -> ()  [unwired: 2 in, 2 out]
                "Auto Start Temp" <- w828
              }
              frame #4 {
              }
            }
          }
        }
        n776 = local read "Auto Start Test"() -> (w799:bool)
        n777 = Not(x=w799) -> (.not. x?=w798:bool)
        n778 = Select(t=Auto_Start_enum."close", s=w798, f=w800) -> (s? t:f=w801:T14)
      }
      frame "Start Stage" {
        w830 = TRUE ("PAUSE")
        n779 = local read "Auto Start Test"() -> (w835:bool)
        n780 = Not(x=w835) -> (.not. x?=w834:bool)
        n781 = Select(t=Auto_Start_enum."close" ("Enum - Selector"), s=w834, f=Auto_Start_enum."Start Stage" ("Enum - Selector")) -> (s? t:f=w831:T14)
        n782 = call "ELAPSED TIMER VI.vi"("RESET"=w830, "PAUSE"=w830) -> ()  [unwired: 7 in, 3 out]
      }
      frame "close" {
        w837 = FALSE ("Heater Button")
        n783 = local write "RUN"(w837) -> ()
        n784 = local write "Heater Button"(w837) -> ()
        n785 = local write "Humidity"(w837) -> ()
        n786 = local write "Auto Start Test"(w837) -> ()
        n787 = property on="Heater Button" class="Bool (strict)"("Val(Sgnl)"=FALSE ("Value (Signaling)")) -> ()  [unwired: 2 in, 2 out]
      }
      frame "Exit" {
      }
    }
    n788 = Wait (ms)(milliseconds to wait=u32 100) -> ()  [unwired: 1 out]
    n789 = local read "Quit"() -> (w733:bool)
  }
  n790 = property on="Service Password Log" class="Str"("Visible"=w21) -> ()  [unwired: 2 in, 2 out]
  n791 = property on="Password 3" class="Clust (strict)"("Visible"=w21) -> ()  [unwired: 2 in, 2 out]
  n792 = while {
    stop <- w866 stop-if-true
    w849 = errorcluster {"status"=FALSE, "code"=0, "source"=""} ("error in (no error) 3")
    # "this loop is for manual report generation"
    n793 = local read "Confirm Measrurement"() -> (w848:bool)
    n794 = case shown="True" w848 {
      selector: w848 -> [_ w956]
      tunnel: errorcluster {"status"=FALSE, "code"=0, "source"=""} ("error in (no error) 3") -> [_ w957]
      tunnel: [_ w955] -> _
      frame False {
      }
      frame True {
        n795 = stacked-sequence {
          tunnel: w957 -> [_ w990 _]
          tunnel: w956 -> [_ _ w1097]
          tunnel: [_ w978 _] -> w955
          frame #0 {
            n796 = String To Path(string="C:\\LAB-IQ\\Image Calibrate v01.dcf") -> (path=w960:path)
            n797 = Open/Create/Replace File ("Open File")(file path (use dialog)=w960) -> (refnum out=w961:refnum<file>)  [unwired: 5 in, 2 out]
            n798 = for {
              N: 4 -> [_]
              tunnel: w961 -> [w967]
              i -> [w963]
              n799 = Read from Text File ("Read File")(file (use dialog)=w967) -> (text=w968:string)  [unwired: 3 in, 3 out]
              n800 = String Subset(string=w968, offset (0)=6, length (rest)=10 ("length (rest)")) -> (substring=w964:string)
              n801 = Fract/Exp String To Number(string=w964) -> (number=w962:dbl)  [unwired: 3 in, 1 out]
              n802 = case shown="3" w963 {
                tunnel: w962 -> [w969 w970 _ w971 _]
                frame 0 {
                  n803 = local write "5x Gain"(w969) -> ()
                }
                frame 1 {
                  n804 = local write "10x Gain"(w970) -> ()
                }
                frame 2 {
                }
                frame 3 {
                  n805 = local write "100x gain"(w971) -> ()
                }
                frame 4, Default {
                }
              }
            }
          }
          frame #1 {
            n806 = local read "TEST STANDARD"() -> (w973:T3)
            n807 = case shown="\"ISO 12156\"" w973 {
              tunnel: ["ASTM D6079" "ISO 12156"] -> w972
              frame "ASTM D6079", Default {
              }
              frame "ISO 12156" {
              }
            }
            n808 = call "IMAGE ANALYSIS.vi"("Enum"=POST_ANALYSIS_ENUM."GET MEASUREMENTS", "error in"=w990) -> ("error out"=w997:errorcluster)  [unwired: 8 in, 1 out]
            n809 = local read "Magnification :"() -> (w983:string)
            n810 = call "Stall Data Flow.vim"("value in"=w997, "milliseconds to wait"=u32 1000) -> ("value out"=w996:errorcluster)  [unwired: 1 out]
            n811 = local read "Test File List :"() -> (w994:string)
            n812 = case shown="\"10x\"" w983 {
              tunnel: [w1033 w1034] -> w981
              frame "5x", Default {
                n813 = local read "5x Gain"() -> (w1033:dbl)
              }
              frame "10x" {
                # "5x"
                n814 = local read "10x Gain"() -> (w1034:dbl)
              }
            }
            n815 = call "IMAGE ANALYSIS.vi"("Enum"=POST_ANALYSIS_ENUM."READ", "error in"=w996) -> ("error out"=w993:errorcluster, "data out"=w984:string)  [unwired: 8 in]
            n816 = Match Pattern(string=w984, regular expression="\"type\": ") -> (after substring=w988:string)  [unwired: 1 in, 3 out]
            n817 = call "IMAGE PATH CREATION PY.vi"("error in (no error)"=w993, "File Name :"=w994) -> ("error out"=w992:errorcluster, "File Path"=w980:path, "File Path String:"=w975:string)  [unwired: 7 in]
            n818 = Match Pattern(string=w988, regular expression=",") -> (before substring=w974:string)  [unwired: 1 in, 3 out]
            n819 = local read "Calibration Tab"() -> (w977:enum32{"Measrument", "Calibrate"})
            n820 = call "Stall Data Flow.vim"("value in"=w992, "milliseconds to wait"=u32 250) -> ("value out"=w976:errorcluster)  [unwired: 1 out]
            n821 = Equal?(x=w974, y="\"rectangle\"") -> (x = y?=w985:bool)
            n822 = case shown="False" w985 {
              tunnel: w984 -> [w1039 w1094]
              tunnel: w981 -> [_ w1085]
              tunnel: cluster{"major":dbl, "minor":dbl, "average":dbl} {"major"=0.0, "minor"=0.0, "average"=0.0} -> [w1037 w1081]
              tunnel: [w1036 w1078] -> w979
              tunnel: w974 -> [w1038 _]
              tunnel: w981 -> [w1035 _]
              frame False {
                n823 = Equal?(x=w1038, y="\"line\"") -> (x = y?=w1040:bool)
                n824 = case shown="True" w1040 {
                  tunnel: w1039 -> [_ w1055]
                  tunnel: w1037 -> [w1042 w1054]
                  tunnel: [w1042 w1052] -> w1036
                  tunnel: w1035 -> [_ w1051]
                  frame False {
                  }
                  frame True {
                    w1050 = 0.0 ("Major Axis")
                    n825 = Match Pattern(string=w1055, regular expression="\"length_px\":") -> (after substring=w1053:string)  [unwired: 1 in, 3 out]
                    n826 = property on="Major Axis" class="DigNum (strict)"("Caption.Text"="") -> ()  [unwired: 2 in, 2 out]
                    n827 = property on="Minor Axis" class="DigNum (strict)"("Caption.Text"="") -> ()  [unwired: 2 in, 2 out]
                    n828 = property on="Average" class="DigNum (strict)"("Caption.Text"="Line") -> ()  [unwired: 2 in, 2 out]
                    n829 = Fract/Exp String To Number(string=w1053, default (0 dbl)=0.0 ("default (0 DBL)")) -> (number=w1049:dbl)  [unwired: 2 in, 1 out]
                    "Pixel Value" <- w1049
                    n830 = Multiply(x=w1049, y=w1051) -> (x*y=w1062:dbl)
                    n831 = Multiply(x=w1062, y=1000.0) -> (x*y=w1045:dbl)
                    n832 = Divide(x=w1045, y=1000.0) -> (x/y=w1048:dbl)
                    n833 = local write "Measurment (mm)"(w1048) -> ()
                    n834 = Bundle By Name(cluster=w1054, "average"=w1045) -> (w1052:cluster{"major":dbl, "minor":dbl, "average":dbl})
                    n835 = Number To Fractional String(number=w1045, precision (6)=i16 1) -> (F-format string=w1044:string)  [unwired: 2 in]
                    n836 = local write "Minor Axis"(w1050) -> ()
                    n837 = local write "Major Axis"(w1050) -> ()
                    n838 = Fract/Exp String To Number(string=w1044) -> (number=w1043:dbl)  [unwired: 3 in, 1 out]
                    n839 = local write "Average"(w1043) -> ()
                  }
                }
              }
              frame True {
                w1082 = 1000.0 ("y")
                w1088 = 0.0 ("default (0 DBL)")
                n840 = Match Pattern(string=w1094, regular expression=" \"width_px\":") -> (after substring=w1092:string)  [unwired: 1 in, 3 out]
                n841 = Match Pattern(string=w1092, regular expression="\"height_px\":") -> (before substring=w1090:string, after substring=w1089:string)  [unwired: 1 in, 2 out]
                n842 = Fract/Exp String To Number(string=w1090, default (0 dbl)=w1088) -> (number=w1087:dbl)  [unwired: 2 in, 1 out]
                n843 = Fract/Exp String To Number(string=w1089, default (0 dbl)=w1088) -> (number=w1086:dbl)  [unwired: 2 in, 1 out]
                n844 = Multiply(x=w1087, y=w1085) -> (x*y=w1084:dbl)
                n845 = Multiply(x=w1086, y=w1085) -> (x*y=w1083:dbl)
                n846 = Multiply(x=w1084, y=w1082) -> (x*y=w1068:dbl)
                n847 = Multiply(x=w1083, y=w1082) -> (x*y=w1066:dbl)
                n848 = Add(x=w1068, y=w1066) -> (x+y=w1080:dbl)
                n849 = property on="Major Axis" class="DigNum (strict)"("Caption.Text"="Major Axis") -> ()  [unwired: 2 in, 2 out]
                n850 = property on="Minor Axis" class="DigNum (strict)"("Caption.Text"="Minor Axis") -> ()  [unwired: 2 in, 2 out]
                n851 = property on="Average" class="DigNum (strict)"("Caption.Text"="Average") -> ()  [unwired: 2 in, 2 out]
                n852 = Divide(x=w1080, y=2.0) -> (x/y=w1064:dbl)
                n853 = Bundle By Name(cluster=w1081, "major"=w1068, "minor"=w1066, "average"=w1064) -> (w1078:cluster{"major":dbl, "minor":dbl, "average":dbl})
                n854 = Number To Fractional String(number=w1066, precision (6)=i16 1) -> (F-format string=w1073:string)  [unwired: 2 in]
                n855 = Number To Fractional String(number=w1064, precision (6)=i16 1) -> (F-format string=w1074:string)  [unwired: 2 in]
                n856 = Number To Fractional String(number=w1068, precision (6)=i16 1) -> (F-format string=w1072:string)  [unwired: 2 in]
                n857 = Fract/Exp String To Number(string=w1073) -> (number=w1065:dbl)  [unwired: 3 in, 1 out]
                n858 = Fract/Exp String To Number(string=w1074) -> (number=w1063:dbl)  [unwired: 3 in, 1 out]
                n859 = Fract/Exp String To Number(string=w1072) -> (number=w1067:dbl)  [unwired: 3 in, 1 out]
                n860 = local write "Major Axis"(w1067) -> ()
                n861 = local write "Average"(w1063) -> ()
                n862 = local write "Minor Axis"(w1065) -> ()
              }
            }
            n863 = case shown="\"Measrument\", Default" w977 {
              tunnel: w980 -> [w1007 _]
              tunnel: w979 -> [w1006 _]
              tunnel: [w1003 w1032] -> w978
              tunnel: w976 -> [w1005 w1032]
              tunnel: w975 -> [w1004 _]
              tunnel: w972 -> [w1002 _]
              frame "Measrument", Default {
                n864 = stacked-sequence {
                  tunnel: w1007 -> [w1025 _]
                  tunnel: w1006 -> [w1023 _]
                  tunnel: w1005 -> [w1021 _]
                  tunnel: w1004 -> [w1020 _]
                  tunnel: [w1015 _] -> w1003
                  tunnel: w1002 -> [w1008 _]
                  frame #0 {
                    n865 = call "IMAGE ANALYSIS.vi"("Enum"=POST_ANALYSIS_ENUM."SAVE IMAGE", "error in"=w1021, "IMAGE FILE PATH"=w1020) -> ("error out"=w1019:errorcluster)  [unwired: 7 in, 1 out]
                    n866 = call "Stall Data Flow.vim"("value in"=w1019, "milliseconds to wait"=u32 1000) -> ("value out"=w1010:errorcluster)  [unwired: 1 out]
                    n867 = local read "Test File List :"() -> (w1027:string)
                    n868 = call "IMAGE ANALYSIS.vi"("Enum"=POST_ANALYSIS_ENUM."MINIMIZE UI", "error in"=w1010) -> ("error out"=w1017:errorcluster)  [unwired: 8 in, 1 out]
                    n869 = Bundle By Name(cluster=T24 {"File Name"="", "Test Method"="", "Operator"="", "Fuel Description"="", "Date and time"=""} ("Main Ref"), "Test Method"=w1008, "File Name"=w1027) -> (w1028:T24)
                    n870 = call "Stall Data Flow.vim"("value in"=w1017, "milliseconds to wait"=u32 1500) -> ("value out"=w1012:errorcluster)  [unwired: 1 out]
                    n871 = call "duf file read.vi"("error in (no error)"=w1012, "Main Ref"=w1028) -> ("error out"=w1026:errorcluster, "Main Ref 2"=w1024:T24)  [unwired: 8 in]
                    n872 = call "DETECTION REPORT for manual.vi"("error in (no error)"=w1026, "return value 3"=w1023, "Image File Path"=w1025, "Main Ref"=w1024) -> ("error out"=w1022:errorcluster)  [unwired: 7 in]
                    n873 = call <vilib>:"Clear Errors.vi"("error in (no error)"=w1022) -> ("error out"=w1013:errorcluster)  [unwired: 5 in, 1 out]
                    n874 = call "IMAGE ANALYSIS.vi"("Enum"=POST_ANALYSIS_ENUM."MINIMIZE UI", "error in"=w1013) -> ("error out"=w1015:errorcluster)  [unwired: 8 in, 1 out]
                  }
                  frame #1 {
                    n875 = local write "Main Tab"(T2."HOME" ("Main Tab")) -> ()
                    n876 = local write "Main Dashboard Buttons"(T1."Home" ("Main Dashboard Buttons")) -> ()
                  }
                }
              }
              frame "Calibrate" {
              }
            }
          }
          frame #2 {
            n877 = Not(x=w1097) -> (.not. x?=w1096:bool)
            n878 = local write "Confirm Measrurement"(w1096) -> ()
            n879 = local read "Calibration Tab"() -> (w1095:enum32{"Measrument", "Calibrate"})
            n880 = case shown="\"Measrument\", Default" w1095 {
              frame "Measrument", Default {
                (unwired) T19."HOME" ("Main Tab")
                n881 = local write "Main Tab"(T2."HOME" ("Main Tab")) -> ()
              }
              frame "Calibrate" {
              }
            }
          }
        }
      }
    }
    n882 = local read "Humidity"() -> (w840:bool)
    n883 = local read "Save Change"() -> (w845:bool)
    n884 = local read "Calibrate"() -> (w846:bool)
    n885 = local read "Auto Start Test"() -> (w841:bool)
    n886 = case shown="True" w846 {
      selector: w846 -> [_ w953]
      frame False {
      }
      frame True {
        n887 = Not(x=w953) -> (.not. x?=w952:bool)
        n888 = local write "Calibrate"(w952) -> ()
        n889 = local write "Calibration Tab"(enum32{"Measrument", "Calibrate"}."Calibrate" ("Calibration Tab")) -> ()
      }
    }
    n890 = case shown="True" w845 {
      selector: w845 -> [_ w897]
      frame False {
      }
      frame True {
        n891 = stacked-sequence {
          tunnel: w897 -> [_ _ _ _ w951]
          frame #0 {
            n892 = call "IMAGE ANALYSIS.vi"("Enum"=POST_ANALYSIS_ENUM."HIDE UI") -> ()  [unwired: 9 in, 2 out]
          }
          frame #1 {
            n893 = local read "100x gain"() -> (w899:dbl)
            n894 = local read "10x Gain"() -> (w900:dbl)
            n895 = local read "5x Gain"() -> (w901:dbl)
            n896 = Number To Fractional String(number=w900, width (-)=i16 4, precision (6)=i16 7) -> (F-format string=w922:string)  [unwired: 1 in]
            n897 = Number To Fractional String(number=0.0, width (-)=i16 4, precision (6)=i16 7) -> (F-format string=w917:string)  [unwired: 1 in]
